vi "Product info.vi"(6 "Info action":T1, 8 "error in (no error)":errorcluster, 10 "Project Code":string, 11 "Part No":string) -> (0 "error out":errorcluster, 2 "Project Code":string, 3 "Part No":string[](array[string]))   [LabVIEW 2017]
uses:
  subVIs/File/Control/Info action.ctl
  Control/Parent path.ctl
  <vilib>/Utility/config.llb/Write Key (String).vi
  <vilib>/Utility/config.llb/Read Key (String).vi
  File.lvlib
  <vilib>/Utility/config.llb/NI_LVConfig.lvlib
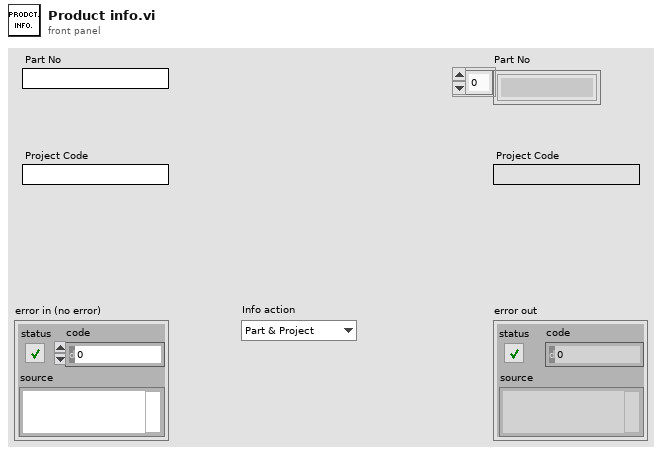
[diagram p1: front panel]
types:
  T1 = typedef "Info action.ctl" = enum16{"Part & Project", "Project Code", "Part No"}
  T2 = typedef "File.lvlib/Parent path.ctl" = enum16{"Project", "Setting", "Log"}
  T3 = typedef "NI_LVConfig.lvlib/Config Data RefNum.ctl" = refnum<k1>
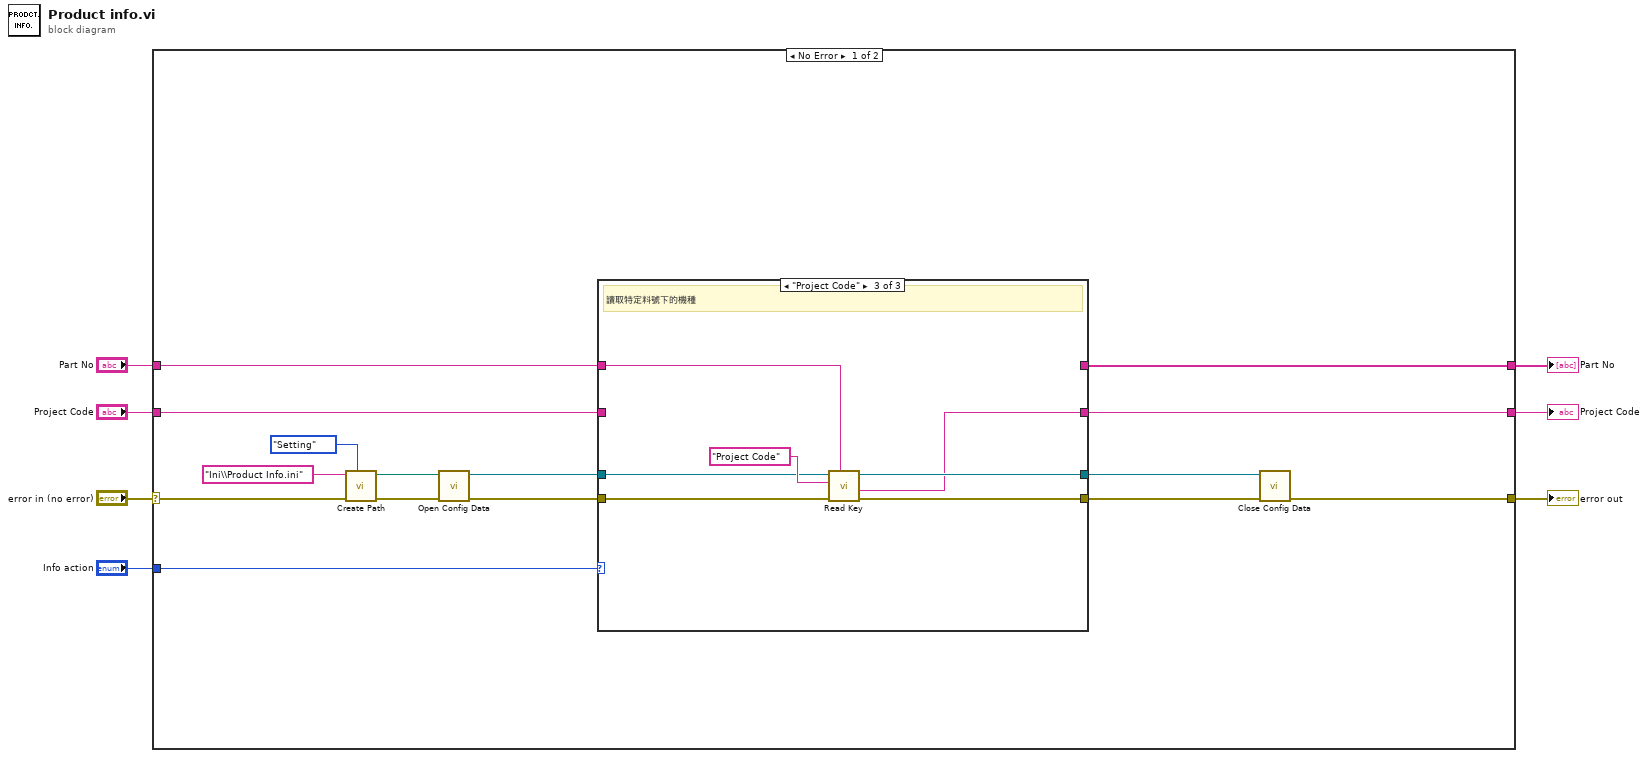
[diagram p0: block diagram]
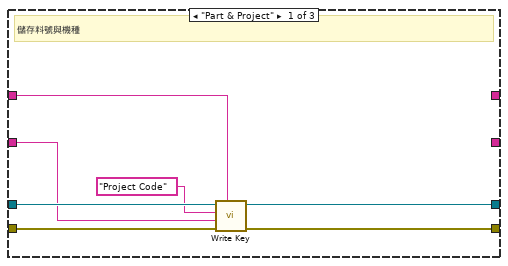
[diagram p2: hidden frame]
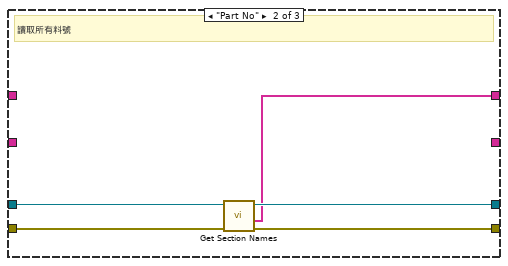
[diagram p3: hidden frame]
diagram:
  n1 = case shown="No Error" "error in (no error)" {
    selector: "error in (no error)" -> [w22 w42]
    tunnel: [w15 w42] -> w6
    tunnel: "Project Code" -> [w13 _]
    tunnel: "Part No" -> [w12 _]
    tunnel: "Info action" -> [w11 _]
    tunnel: [w10 _] -> w3
    tunnel: [w9 _] -> w1
    frame No Error {
      n2 = call "Create Path.vi"("Parent path"=Parent_path."Setting", "error in (no error)"=w22, "Directory"="Ini\\Product Info.ini") -> ("error out"=w21:errorcluster, "Path"=w18:path)  [unwired: 7 in]
      n3 = call <vilib>:"Open Config Data.vi"("error in (no error)"=w21, "configuration file path"=w18) -> ("error out"=w19:errorcluster, "refnum"=w16:T3)  [unwired: 7 in, 1 out]
      n4 = case shown="\"Project Code\"" w11 {
        tunnel: w19 -> [w29 w34 w41]
        tunnel: [w28 w33 w40] -> w17
        tunnel: w16 -> [w27 w32 w35]
        tunnel: [w26 w31 w39] -> w14
        tunnel: w13 -> [w25 _ _]
        tunnel: w12 -> [w24 _ w38]
        tunnel: [_ _ w36] -> w10
        tunnel: [_ w30 _] -> w9
        frame "Part & Project" {
          # "儲存料號與機種"
          n5 = call-poly <vilib>:"Write Key.vi"("section"=w24, "error in (no error)"=w29, "value"=w25, "key"="Project Code", "refnum"=w27) -> ("error out"=w28:errorcluster, "refnum out"=w26:T3)  [unwired: 4 in, 1 out]
        }
        frame "Part No" {
          # "讀取所有料號"
          n6 = call <vilib>:"Get Section Names.vi"("error in (no error)"=w34, "refnum"=w32) -> ("error out"=w33:errorcluster, "section names"=w30:string[], "refnum out"=w31:T3)  [unwired: 7 in]
        }
        frame "Project Code" {
          # "讀取特定料號下的機種"
          n7 = call-poly <vilib>:"Read Key.vi"("section"=w38, "error in (no error)"=w41, "key"="Project Code", "refnum"=w35) -> ("error out"=w40:errorcluster, "value"=w36:string, "refnum out"=w39:T3)  [unwired: 4 in, 1 out]
        }
      }
      n8 = call <vilib>:"Close Config Data.vi"("error in (no error)"=w17, "refnum"=w14) -> ("error out"=w15:errorcluster)  [unwired: 8 in, 1 out]
    }
    frame Error {
    }
  }
  "error out" <- w6
  "Project Code" <- w3
  "Part No" <- w1
